vi "action.vi"(0 "HGF_ThreadTaskLoop":refnum<class "HGF_TaskLoop.lvclass">, 5 "error in (no error)":errorcluster, 8 "HGF_ThreadWorker":refnum<class "HGF_ThreadWorker.lvclass">) -> (10 "dup HGF_ThreadWorker":refnum<class "HGF_ThreadWorker.lvclass">, 14 "dup HGF_ThreadTaskLoop":refnum<class "HGF_TaskLoop.lvclass">, 19 "error out":errorcluster)   [LabVIEW 2014, in "HGF_BaseClasses.lvlib" / "HGF_TaskLoop.lvclass"]
doc: "This is a dynamic dispatch VI that is called from Visitor.visit(). It will call member VIs of Visitable to perform the requested action which means: calling public methods of Visitable child class.\n\n<B>Hint:</B> This method is abstract and need to be implemented by child classes."
uses:
  HGF_TaskLoop.lvclass
  HGF_ThreadTask/HGF_ThreadTask.lvclass
  HGF_Visitor/HGF_Visitor.lvclass
  HGF_Stop/HGF_Stop.lvclass
  HGF_ThreadWorker/HGF_ThreadWorker.lvclass
  HGF_Event/HGF_Event.lvclass
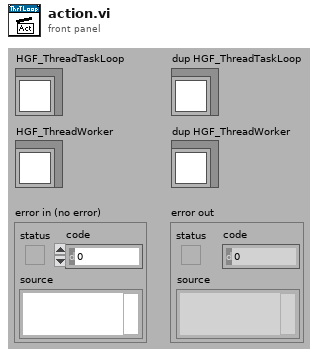
[diagram p1: front panel]
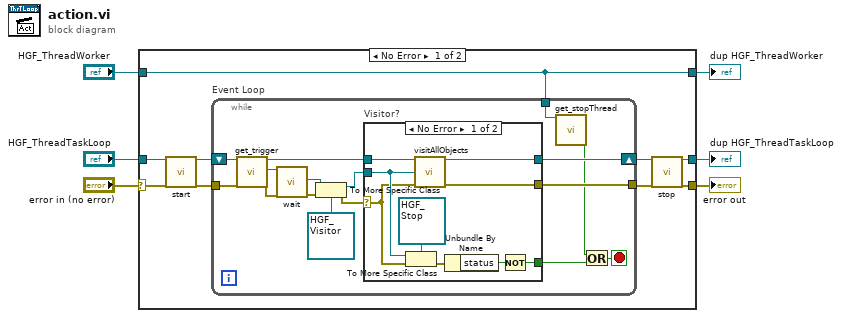
[diagram p0: block diagram]
diagram:
  n1 = case shown="No Error" "error in (no error)" {
    selector: "error in (no error)" -> [w13 w44]
    tunnel: "HGF_ThreadTaskLoop" -> [w15 w45]
    tunnel: [w10 w45] -> w2
    tunnel: [w8 w44] -> w1
    tunnel: [w7 w43] -> w3
    tunnel: "HGF_ThreadWorker" -> [w7 w43]
    frame No Error {
      n2 = call "start.vi"("HGF_TaskLoop in"=w15, "error in (no error)"=w13) -> ("HGF_TaskLoop out"=w14:refnum<class "HGF_TaskLoop.lvclass">, "error out"=w12:errorcluster)  [unwired: 16 in]
      n3 = while "Event Loop" {
        tunnel: [w19] -> w9
        shift-right: [w20] -> w11
        shift-left: w14 -> [w29]
        tunnel: w12 -> [w27]
        tunnel: w7 -> [w18]
        stop <- w17 stop-if-true
        n4 = call "get_trigger.vi"("HGF_ThreadTask"=w29, "error in (no error)"=w27) -> ("dup HGF_ThreadTask"=w28:refnum<class "HGF_TaskLoop.lvclass">, "trigger"=w25:refnum<class "HGF_Event.lvclass">, "error out"=w26:errorcluster)  [unwired: 15 out]
        n5 = call-dynamic "wait.vi"("HGF_Event"=w25, "error in (no error)"=w26) -> ("Object"=w30:refnum<class>, "error out"=w31:errorcluster)  [unwired: 2 in, 14 out]
        n6 = To More Specific Class(target class=refnum<class "HGF_Visitor.lvclass"> refnum ("HGF_BaseClasses.lvlib:HGF_Visitor.lvclass"), reference=w30, error in=w31) -> (specific class reference=w24:refnum<class "HGF_Visitor.lvclass">, error out=w22:errorcluster)
        n7 = case "Visitor?" shown="No Error" w22 {
          selector: w22 -> [w34 w41]
          tunnel: [w32 w41] -> w19
          tunnel: w28 -> [w35 w42]
          tunnel: [w33 w42] -> w20
          tunnel: w24 -> [w36 _]
          tunnel: [w37 _] -> w21
          frame No Error {
            n8 = To More Specific Class(target class=refnum<class "HGF_Stop.lvclass"> refnum ("HGF_BaseClasses.lvlib:HGF_Stop.lvclass"), reference=w36, error in=w34) -> (error out=w39:errorcluster)  [unwired: 1 out]
            n9 = call-dynamic "visitAllObjects.vi"("HGF_ThreadTask"=w35, "HGF_Visitor"=w36, "error in (no error)"=w34) -> ("dup HGF_ThreadTask"=w33:refnum<class "HGF_TaskLoop.lvclass">, "error out"=w32:errorcluster)  [unwired: 11 out]
            n10 = Unbundle By Name(w39) -> ("status"=w38:bool)
            n11 = Not(x=w38) -> (.not. x?=w37:bool)
          }
          frame Error {
          }
        }
        n12 = call "get_stopThread.vi"("HGF_ThreadWorker"=w18) -> ("stopThread"=w16:bool)  [unwired: 16 in, 2 out]
        n13 = Or(x=w16, y=w21) -> (x .or. y?=w17:bool)
      }
      n14 = call "stop.vi"("HGF_TaskLoop in"=w11, "error in (no error)"=w9) -> ("HGF_TaskLoop out"=w10:refnum<class "HGF_TaskLoop.lvclass">, "error out"=w8:errorcluster)  [unwired: 16 in]
    }
    frame Error {
    }
  }
  "error out" <- w1
  "dup HGF_ThreadTaskLoop" <- w2
  "dup HGF_ThreadWorker" <- w3
